vi "requestStatus.vi"(8 "error in (no error)":errorcluster, 11 "CameraAcquisitor in":refnum<class "CameraAcquisitor.lvclass">) -> (0 "error out":errorcluster, 2 "String":string, 3 "CameraAcquisitor out":refnum<class "CameraAcquisitor.lvclass">)   [LabVIEW 2011, in "Hardware.lvlib" / "Channels.lvlib" / "CameraAcquisitor.lvclass"]
uses:
  CameraAcquisitor.lvclass
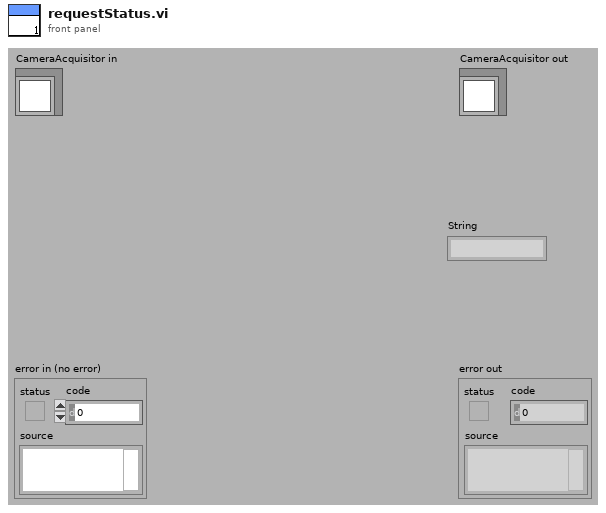
[diagram p1: front panel]
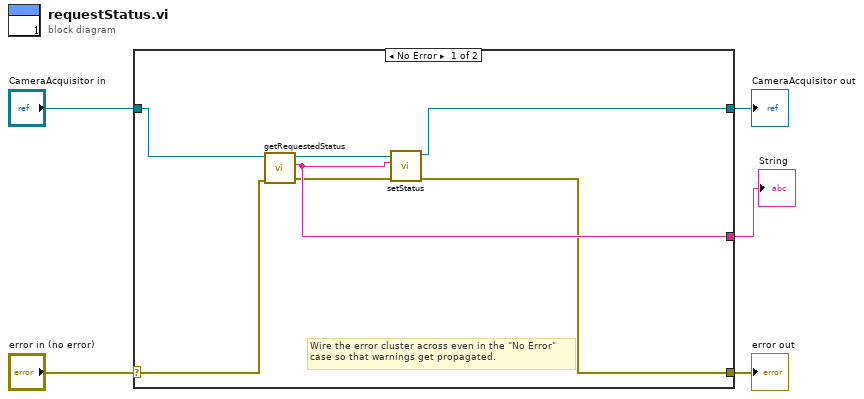
[diagram p0: block diagram]
diagram:
  n1 = case shown="No Error" "error in (no error)" {
    selector: "error in (no error)" -> [w11 w14]
    tunnel: [w6 w14] -> w4
    tunnel: [w7 w13] -> w2
    tunnel: "CameraAcquisitor in" -> [w12 w13]
    tunnel: [w10 _] -> w1
    frame No Error {
      # "Wire the error cluster across even in the \"No Error\"\ncase so that warnings get propagated."
      n2 = call-dynamic "getRequestedStatus.vi"("error in (no error)"=w11, "CameraAcquisitor in"=w12) -> ("error out"=w9:errorcluster, "String"=w10:string, "CameraAcquisitor out"=w8:refnum<class "CameraAcquisitor.lvclass">)  [unwired: 7 in]
      n3 = call-dynamic "setStatus.vi"("error in (no error)"=w9, "Status"=w10, "CameraAcquisitor.lvclass in"=w8) -> ("error out"=w6:errorcluster, "CameraAcquisitor.lvclass out"=w7:refnum<class "CameraAcquisitor.lvclass">)  [unwired: 7 in]
    }
    frame Error {
    }
  }
  "error out" <- w4
  "CameraAcquisitor out" <- w2
  "String" <- w1
